vi "ClientCode.vi"(8 "error in (no error)":errorcluster, 10 "Creator":refnum<class "Creator.lvclass">, 11 "FactoryMethodDemo in":refnum<class "FactoryMethodDemo.lvclass">) -> (0 "error out":errorcluster, 3 "FactoryMethodDemo out":refnum<class "FactoryMethodDemo.lvclass">)   [LabVIEW 2020, in "FactoryMethod.lvlib" / "FactoryMethodDemo.lvclass"]
uses:
  FactoryMethodDemo.lvclass
  Creator/Creator.lvclass
  Support/Class/ConsoleOutput.lvclass
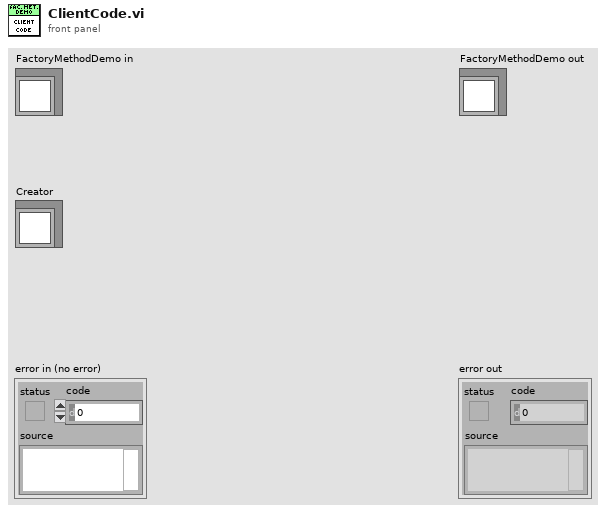
[diagram p1: front panel]
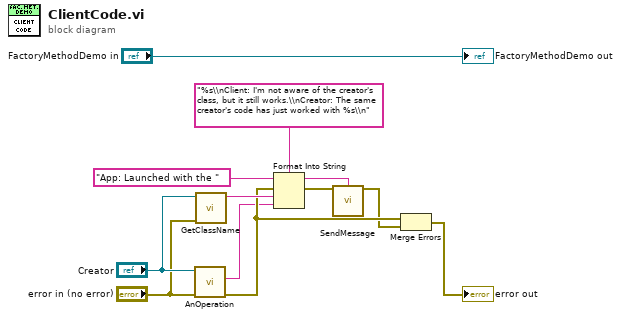
[diagram p0: block diagram]
diagram:
  n1 = call "AnOperation.vi"("error in (no error)"="error in (no error)", "Creator in"="Creator") -> ("error out"=w5:errorcluster, "ResultString"=w3:string)  [unwired: 7 in, 1 out]
  n2 = call "GetClassName.vi"("error in (no error)"="error in (no error)", "object"="Creator") -> ("Class Name"=w6:string)  [unwired: 8 in, 1 out]
  n3 = Format Into String(format string="%s\\nClient: I'm not aware of the creator's class, but it still works.\\nCreator: The same creator's code has just worked with %s\\n", initial string="App: Launched with the " ("Message"), error in=w5, w6, w3) -> (resulting string=w1:string, error out=w10:errorcluster)
  n4 = call "SendMessage.vi"("Message"=w1, "error in (no error)"=w10) -> ("error out"=w2:errorcluster)  [unwired: 13 in]
  n5 = Merge Errors(w5, w2) -> (→"error out":errorcluster)
  "FactoryMethodDemo out" <- "FactoryMethodDemo in"
